vi "看二值化.vi"(8 "error in (no error)":errorcluster, 10 "ROI Descriptor":T1 {"Contours"."Type" items=["No Selection", "Point", "Line", "Rectangle", "Oval", "Polygon", "Freehand Region", "Annulus", "Unused2", "Unused3", "Broken Line", "Freehand Line", "Rotated Rectangle"]}, 11 "Image In":T2(plugin-control)) -> (0 "error out":errorcluster, 1 "Mean":sgl format="%#.2f", 2 "Histogram":T3(graph), 3 "Image Out":T2, 4 "Standard Deviation":sgl format="%#.2f")   [LabVIEW 2015]
doc: "This example shows how to compute the histogram of an image or a region in the image. This example also shows how to set up and use the display tools to select and work on different regions in the image interactively."
uses:
  <vilib>/vision/Image Controls.llb/IMAQ Image.ctl
  <vilib>/vision/NI_Vision_Development_Module.lvlib
panel:
  # "Overview: Demonstrates how to use the IMAQ Histogram function with a mask to return histogram information about the portion of the image in a Region of Interest (ROI).\nRequirements: Vision Development Software.\nInstructions:\n1. Run the VI.\n2. Draw a ROI in the image by left clicking, hold left mouse button down, drag the mouse across the image, and release the mouse button."
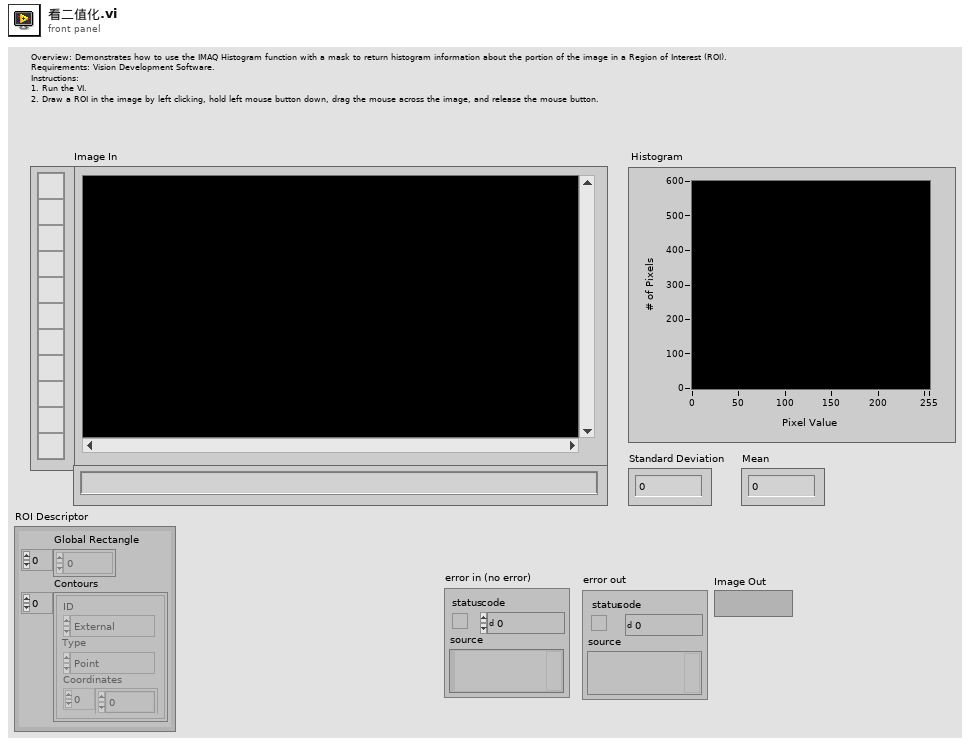
[diagram p1: front panel]
types:
  T1 = typedef "ROI Descriptor" = cluster{"Global Rectangle":i32[], "Contours":cluster{"ID":enum32{"External", "Internal"}, "Type":u32, "Coordinates":i32[]}[]}
  T2 = typedef "IMAQ Image.ctl" = refnum<image>
  T3 = cluster{"Starting Value":sgl, "Incremental Value":sgl, "Histogram":u32[]}
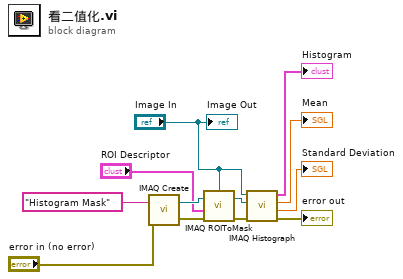
[diagram p0: block diagram]
diagram:
  n1 = call "IMAQ Create"("Image Name"="Histogram Mask", "error in (no error)"="error in (no error)") -> ("New Image"=w11:T2, "error out"=w10:errorcluster)  [unwired: 3 in]
  n2 = call "IMAQ ROIToMask"("error in (no error)"=w10, "ROI Descriptor"="ROI Descriptor", "Image"=w11, "Image Model"="Image In") -> ("error out"=w6:errorcluster, "Image Out"=w7:T2)  [unwired: 2 in, 1 out]
  n3 = call "IMAQ Histograph"("error in (no error)"=w6, "Image Mask"=w7, "Image"="Image In") -> ("error out"=→"error out":errorcluster, "Standard  Deviation"=→"Standard Deviation":sgl, "Mean Value"=→"Mean":sgl, "Histogram Graph"=→"Histogram":T3)  [unwired: 5 in]
  "Image Out" <- "Image In"
